vi "ALapp_P_term.vi"(1 "P Term Gain":dbl, 3 "Error":dbl) -> (0 "P Term":dbl)   [LabVIEW 2011]
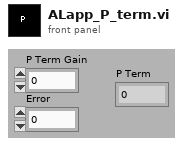
[diagram p1: front panel]
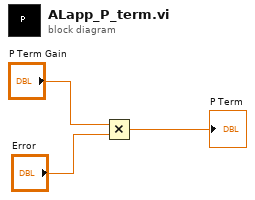
[diagram p0: block diagram]
diagram:
  n1 = Multiply(x="P Term Gain", y="Error") -> (x*y=→"P Term":dbl)
